vi "TIO Data Stream Log.vi"(8 "Data Out":T3, 9 "TIO State":T2={"Awaiting REP"=FALSE, "REQ ID"=500, "streams in"=[], "sources"=[], "timebases"=[]}, 10 "Data Out":T1(array[cluster])=[{"Name"="gmr", "Waveform"={"start"=0.0, "dt"=1.0, "Timeseries"=[[-1045203.625, 2103369.25, -524451.0625]]}}, {"Name"="accel", "Waveform"={"start"=0.0, "dt"=1.0, "Timeseries"=[[0.4673272967338562, -9.214466094970703, -3.09728741645813]]}}, {"Name"="gyro", "Waveform"={"start"=0.0, "dt"=1.0, "Timeseries"=[[0.019417261704802513, 0.00881516095250845, 0.006293708924204111]]}}, {"Name"="bar", "Waveform"={"start"=0.0, "dt"=1.0, "Timeseries"=[[0.0]]}}, {"Name"="therm", "Waveform"={"start"=0.0, "dt"=1.0, "Timeseries"=[[0.0]]}}], 11 "Log to file":path) -> ()   [LabVIEW 2020]
uses:
  <vilib>/Utility/file.llb/Write Delimited Spreadsheet (DBL).vi
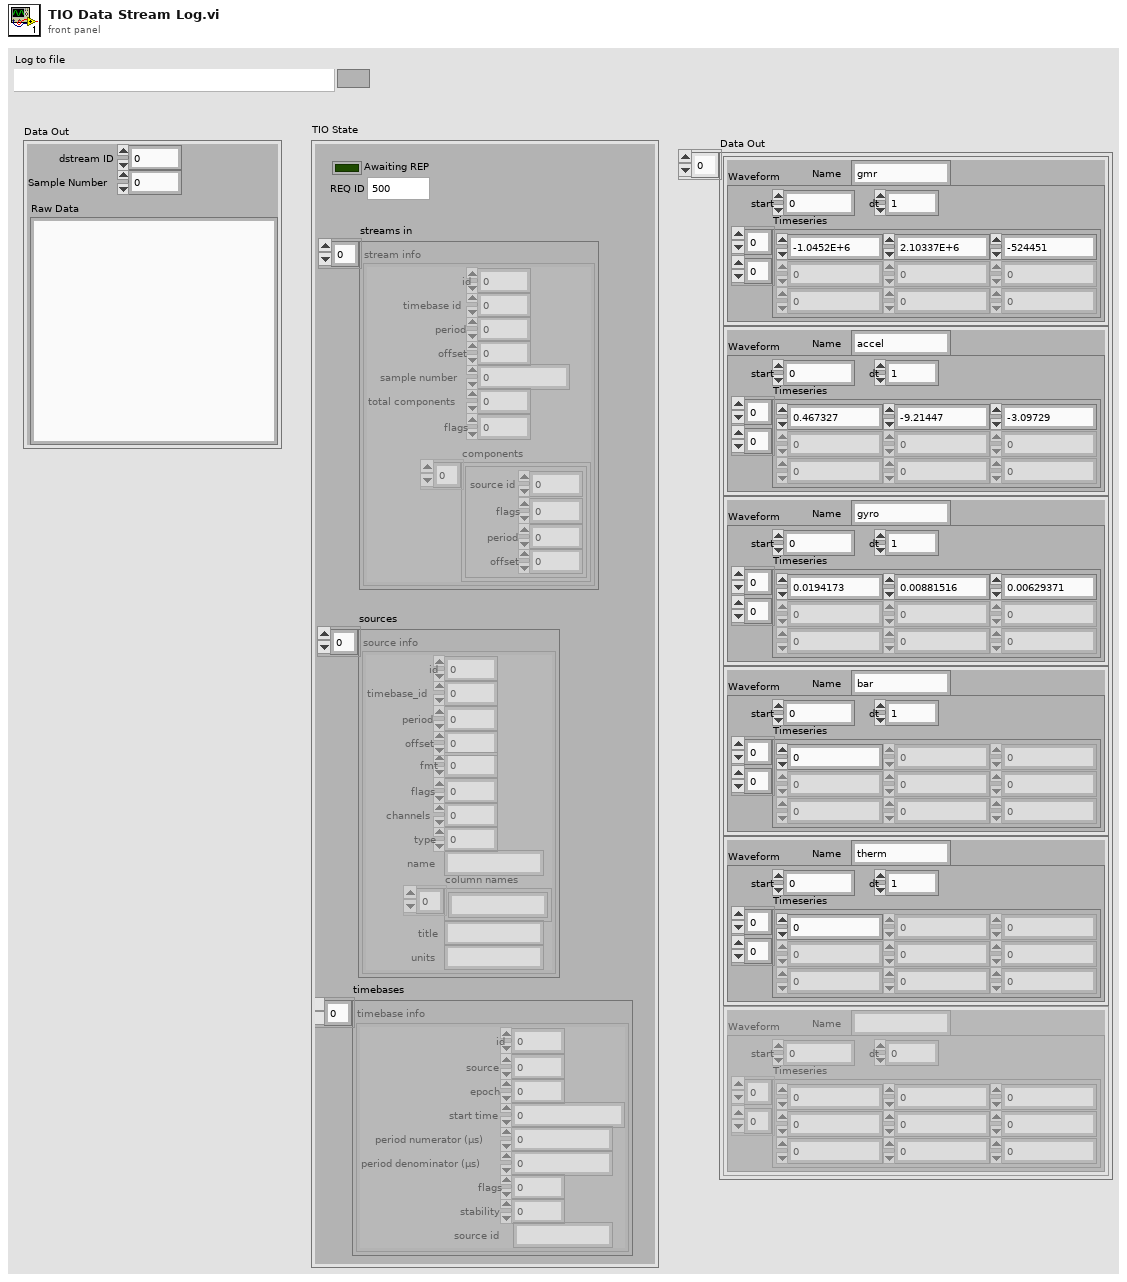
[diagram p1: front panel]
types:
  T1 = cluster{"Name":string, "Waveform":cluster{"start":dbl, "dt":dbl, "Timeseries":dbl[][]}}[]
  T2 = cluster{"Awaiting REP":bool, "REQ ID":u32, "streams in":cluster{"id":u16, "timebase id":u16, "period":u32, "offset":u32, "sample number":u64, "total components":u16, "flags":u16, "components":cluster{"source id":u16, "flags":u16, "period":u32, "offset":u32}[]}[], "sources":cluster{"id":u16, "timebase_id":u16, "period":u32, "offset":u32, "fmt":i32, "flags":u16, "channels":u16, "type":u8, "name":string, "column names":string[], "title":string, "units":string}[], "timebases":cluster{"id":u16, "source":u8, "epoch":u8, "start time":u64, "period numerator (µs)":u32, "period denominator (µs)":u32, "flags":u32, "stability":sgl, "source id":string}[]}
  T3 = cluster{"dstream ID":u16, "Sample Number":u32, "Raw Data":string}
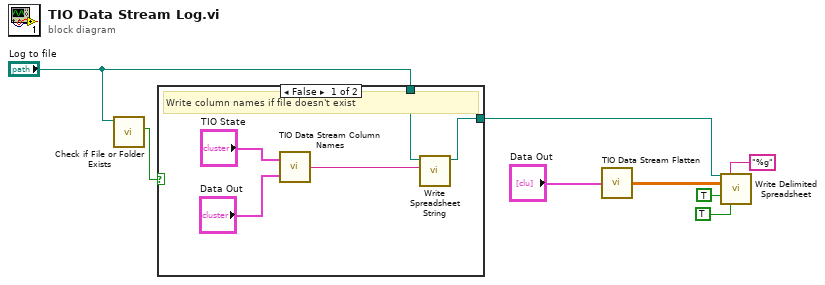
[diagram p0: block diagram]
diagram:
  n1 = call <vilib>:"Check if File or Folder Exists.vi"("path"="Log to file") -> ("file or folder exists?"=w3:bool)  [unwired: 8 in, 2 out]
  n2 = case shown="False" w3 {
    tunnel: "Log to file" -> [w10 w14]
    tunnel: [w9 w14] -> w1
    frame False {
      # "Write column names if file doesn't exist"
      n3 = call <instrlib>:"TIO Data Stream Column Names.vi"("Raw Data"="Data Out", "TIO State"="TIO State") -> ("String"=w11:string)
      n4 = call <vilib>:"Write Spreadsheet String.vi"("spreadsheet string"=w11, "file path (dialog if empty)"=w10) -> ("path"=w9:path)  [unwired: 8 in, 1 out]
    }
    frame True {
    }
  }
  n5 = call <instrlib>:"TIO Data Stream Flatten.vi"("Data Out"="Data Out") -> ("Flattened Array"=w8:dbl[][])
  n6 = call-poly <vilib>:"Write Delimited Spreadsheet.vi"("file path (dialog if empty)"=w1, "format (%.3f)"="%g", "2D data"=w8, "append to file? (new file:F)"=TRUE ("append to file? (F)"), "transpose? (no:F)"=TRUE ("transpose? (F)")) -> ()  [unwired: 9 in, 2 out]
